vi "Async.OnDoubleClickRuntime2.vi"(0 "XRef":T8, 1 "Point":T6, 2 "Mouse Mods":T4, 3 "State In":T1) -> ()   [LabVIEW 2015, in "Async.xnode"]
uses:
  Async.xnode
  <vilib>/XNodeSupport/XNodeXNodeRef.ctl
  <vilib>/XNodeSupport/XNodePoint.ctl
  <vilib>/XNodeSupport/XNodeInt.ctl
  <vilib>/XNodeSupport/XNodeMouseMods.ctl
  <vilib>/XNodeSupport/XNodeBool.ctl
  State.ctl
  <vilib>/Utility/miscctls.llb/LVRectTypeDef.ctl
  <vilib>/picture/picture.llb/imagedata.ctl
  <vilib>/XNodeSupport/NI_XNodeSupport.lvlib
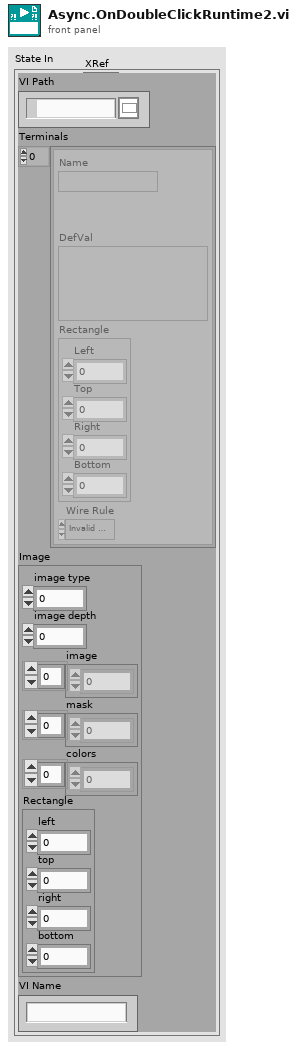
[diagram p1: front panel]
types:
  T1 = typedef "Async.xnode/State.ctl" = cluster{"VI Path":path, "Terminals":cluster{"Name":string, "DefVal":variant, "Rectangle":T2, "Wire Rule":enum16{"Invalid Wire Rule", "Required", "Recommended", "Optional", "Dynamic Dispatch"}}[], "Image":T3, "VI Name":string}
  T2 = typedef "LVRectTypeDef.ctl" = cluster{"Left":i16, "Top":i16, "Right":i16, "Bottom":i16}
  T3 = typedef "imagedata.ctl" = cluster{"image type":i32, "image depth":i32, "image":u8[], "mask":u8[], "colors":u32[], "Rectangle":cluster{"left":i16, "top":i16, "right":i16, "bottom":i16}}
  T4 = typedef "NI_XNodeSupport.lvlib/XNodeMouseMods.ctl" = cluster{"Shift?":T5, "Menu?":T5, "Alt?":T5}
  T5 = typedef "NI_XNodeSupport.lvlib/XNodeBool.ctl" = bool
  T6 = typedef "NI_XNodeSupport.lvlib/XNodePoint.ctl" = cluster{"H":T7, "V":T7}
  T7 = typedef "NI_XNodeSupport.lvlib/XNodeInt.ctl" = i32
  T8 = typedef "NI_XNodeSupport.lvlib/XNodeXNodeRef.ctl" = refnum<vi>
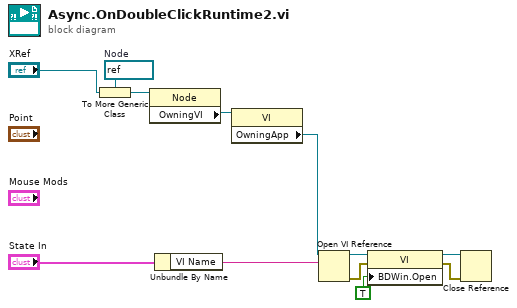
[diagram p0: block diagram]
diagram:
  w8 = refnum<vi> refnum  # Node
  n1 = To More Generic Class(target class=w8, reference="XRef") -> (generic class reference=w7:refnum<vi>)
  n2 = property class="Node"(reference=w7) -> ("OwningVI"=w6:refnum<vi>)  [unwired: 1 in, 2 out]
  n3 = Unbundle By Name("State In") -> ("VI Name"=w10:string)
  n4 = property class="VI"(reference=w6) -> ("OwningApp"=w5:refnum<vi>)  [unwired: 1 in, 2 out]
  n5 = Open VI Reference(application reference (local)=w5, vi path=w10) -> (vi reference=w12:refnum<vi>, error out=w11:errorcluster)  [unwired: 4 in]
  n6 = property class="VI"(reference=w12, error in=w11, "BDWin.Open"=TRUE ("Block Diagram Window:Open")) -> (reference out=w3:refnum<vi>, error out=w4:errorcluster)
  n7 = Close Reference(reference=w3, error in (no error)=w4) -> ()  [unwired: 1 out]
